vi "SetPort.vi"(8 "error in (no error)":errorcluster, 9 "Value":u8, 10 "Port":u8, 11 "Cypress CY8CKIT-059 in":refnum<class "Cypress CY8CKIT-059.lvclass">) -> (0 "error out":errorcluster, 3 "Cypress CY8CKIT-059 out":refnum<class "Cypress CY8CKIT-059.lvclass">)   [LabVIEW 2020, in "Cypress CY8CKIT-059.lvclass"]
doc: "Set a value on a port on the target device."
uses:
  Cypress CY8CKIT-059.lvclass
  Controls/Device Command Code.ctl
  Controls/Device Code.ctl
  Cypress CY8CKIT-059.lvclass/Cypress CY8CKIT-059.ctl
  e83fd593-0d5c-4f49-a376-e4e40c5aca9f.vi
  Read Serial Port.vi
  Write Serial Port.vi
  <vilib>/Utility/error.llb/Error Cluster From Error Code.vi
  <vilib>/ErrorRing/Error Ring.xnode
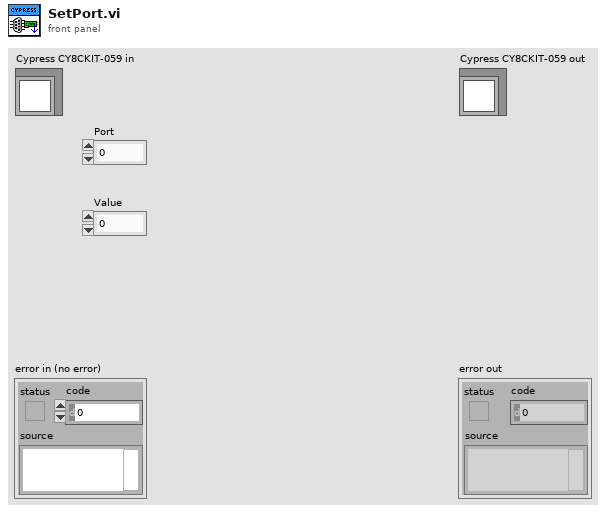
[diagram p1: front panel]
types:
  T1 = typedef "Device Code.ctl" = string
  T2 = typedef "Device Command Code.ctl" = string
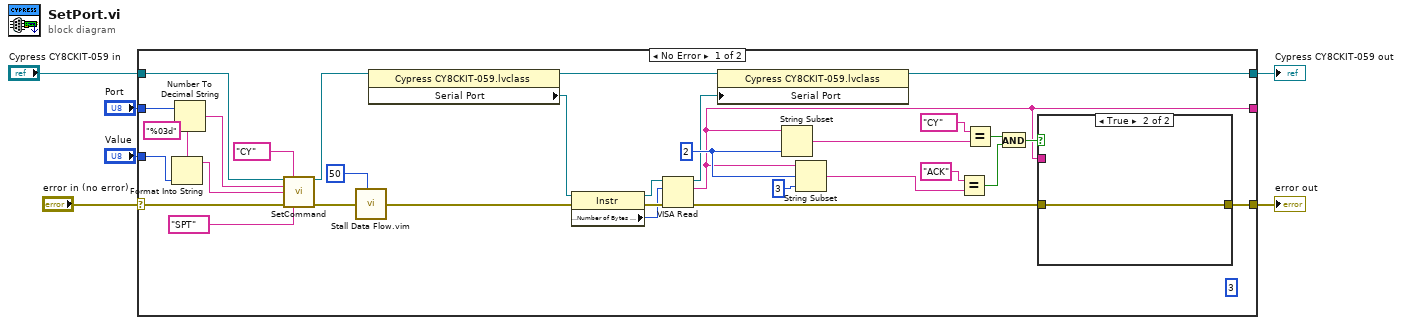
[diagram p0: block diagram]
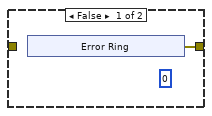
[diagram p2: hidden frame]
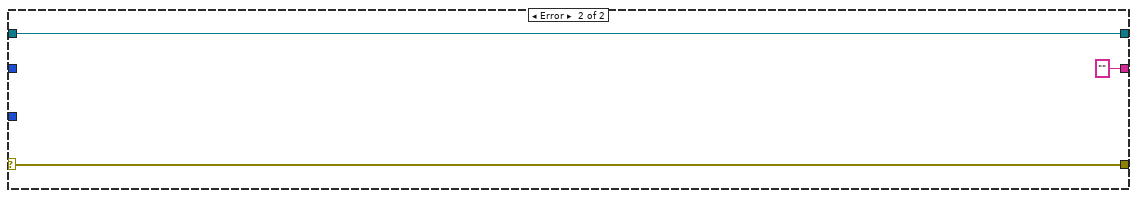
[diagram p3: hidden frame]
diagram:
  n1 = case shown="No Error" "error in (no error)" {
    selector: "error in (no error)" -> [w38 w48]
    tunnel: [w22 w48] -> w2
    tunnel: [w18 w46] -> w3
    tunnel: "Port" -> [w35 _]
    tunnel: [w12 "" ("read buffer")] -> _
    tunnel: "Value" -> [w9 _]
    tunnel: "Cypress CY8CKIT-059 in" -> [w10 w46]
    frame No Error {
      (unwired) 3 ("length (rest)")
      w27 = 2 ("length (rest)")
      n2 = Format Into String(format string="%03d", w9) -> (resulting string=w8:string)  [unwired: 2 in, 1 out]
      n3 = Number To Decimal String(number=w35) -> (decimal integer string=w34:string)  [unwired: 1 in]
      n4 = call-dynamic "SetCommand.vi"("Cypress CY8CKIT-059 in"=w10, "Device Code"=T1 "CY", "Parameter 1"=w34, "Parameter 2"=w8, "error in (no error)"=w38, "Command Code"=T2 "SPT") -> ("Cypress CY8CKIT-059 out"=w33:refnum<class "Cypress CY8CKIT-059.lvclass">, "error out"=w15:errorcluster)  [unwired: 8 in]
      n5 = call "Stall Data Flow.vim"("value in"=w15, "milliseconds to wait"=u32 50) -> ("value out"=w14:errorcluster)  [unwired: 1 out]
      n6 = property class="Cypress CY8CKIT-059.lvclass"(reference=w33) -> (reference out=w19:refnum<class "Cypress CY8CKIT-059.lvclass">, "Serial Port"=w32:refnum<visa-resource-name>)  [unwired: 1 in, 1 out]
      n7 = property class="Instr"(reference=w32, error in=w14) -> (reference out=w30:refnum<visa-resource-name>, error out=w31:errorcluster, "Serial Settings:Number of Bytes at Serial Port"=w29:u32)
      n8 = VISA Read(VISA resource name=w30, byte count=w29, error in (no error)=w31) -> (VISA resource name out=w17:refnum<visa-resource-name>, read buffer=w12:string, error out=w23:errorcluster)  [unwired: 1 out]
      n9 = property class="Cypress CY8CKIT-059.lvclass"(reference=w19, "Serial Port"=w17) -> (reference out=w18:refnum<class "Cypress CY8CKIT-059.lvclass">)  [unwired: 1 in, 1 out]
      n10 = String Subset(string=w12, length (rest)=w27) -> (substring=w20:string)  [unwired: 1 in]
      n11 = String Subset(string=w12, offset (0)=w27, length (rest)=3 ("length (rest)")) -> (substring=w28:string)
      n12 = Equal?(x="ACK", y=w28) -> (x = y?=w25:bool)
      n13 = Equal?(x=T1 "CY" ("Device Code"), y=w20) -> (x = y?=w21:bool)
      n14 = And(x=w21, y=w25) -> (x .and. y?=w24:bool)
      n15 = case shown="True" w24 {
        tunnel: w23 -> [_ w45]
        tunnel: [w39 w45] -> w22
        tunnel: w12 -> [_ _]
        frame False {
          (unwired) u8 0
          n16 = xnode "Error Ring"() -> ("error out"=w39:errorcluster)
        }
        frame True {
        }
      }
    }
    frame Error {
    }
  }
  "error out" <- w2
  "Cypress CY8CKIT-059 out" <- w3
